vi "Daq_withRPM.vi"() -> ()   [LabVIEW 2019]
panel:
  in  "Salvar Ensaio":path
  out "RPM Atual":i32
  in  "Tempo de transição (s)":u32=2000
  out "Running":bool=TRUE
  in  "Parar Ensaio":bool
  in  "Tempo por RPM (min)":dbl
  in  "configuração de porta":T1={"Serial VCC"="", "timeout"=2, "baud rate"=600, "flow control"=0, "data bits"=8, "parity"=enum."None", "stop bits"=10, "termination char"=FALSE} {"stop bits" items=["1.0"=10, "1.5"=15, "2.0"=20]; "flow control" items=["None", "XON/XOFF", "RTS/CTS", "XON/XOFF & RTS/CTS", "DTR/DSR", "XON/XOFF & DTR/DSR"]}
  out "Grafico Aceleração":dynamicdata(graph)
  in  "Start button":bool
  in  "Passo de RPM":i32
  in  "Máximo RPM":i32
  in  "Mínimo RPM":i32
  # "Ensaio de Vibração"
  # "Configuração"
  # "Rodando"
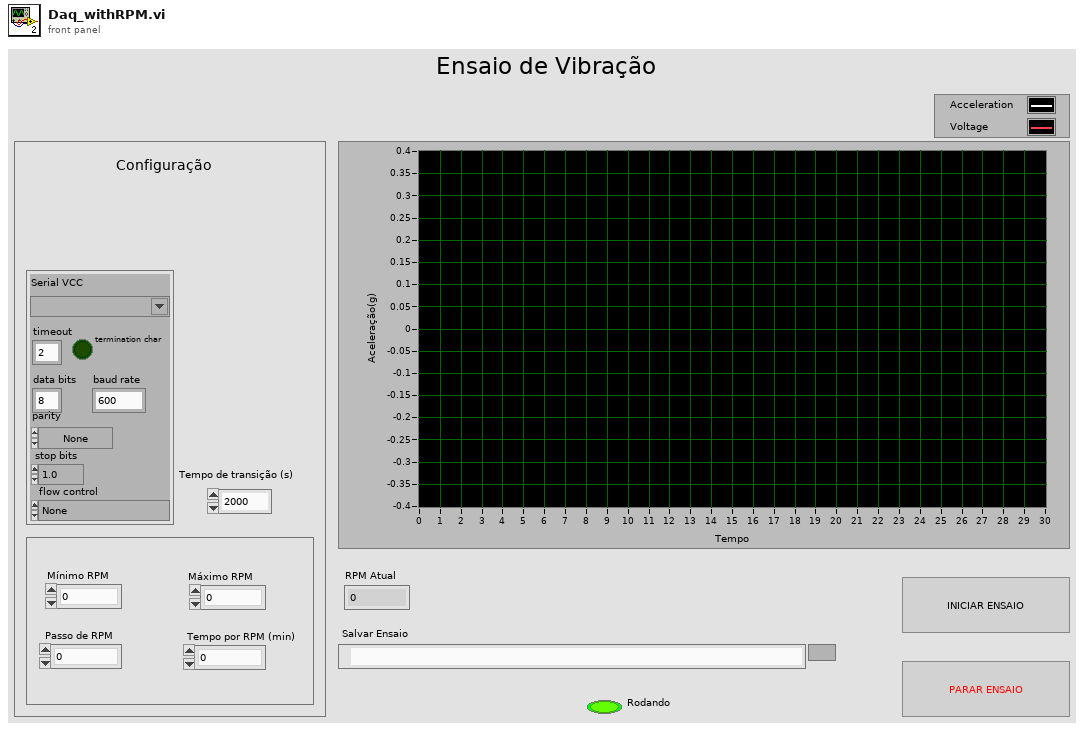
[diagram p1: front panel]
types:
  T1 = cluster{"Serial VCC":refnum<visa-resource-name>, "timeout":u32, "baud rate":u32, "flow control":u16, "data bits":u16, "parity":enum16{"None", "Odd", "Even", "Mark", "Space"}, "stop bits":u16, "termination char":bool}
  T2 = enum16{"Start Comm.", "End Comm.", "Wait", "Send Static Message", "Set Speed", "Set PWM Mode", "Set PWM Frequency"}
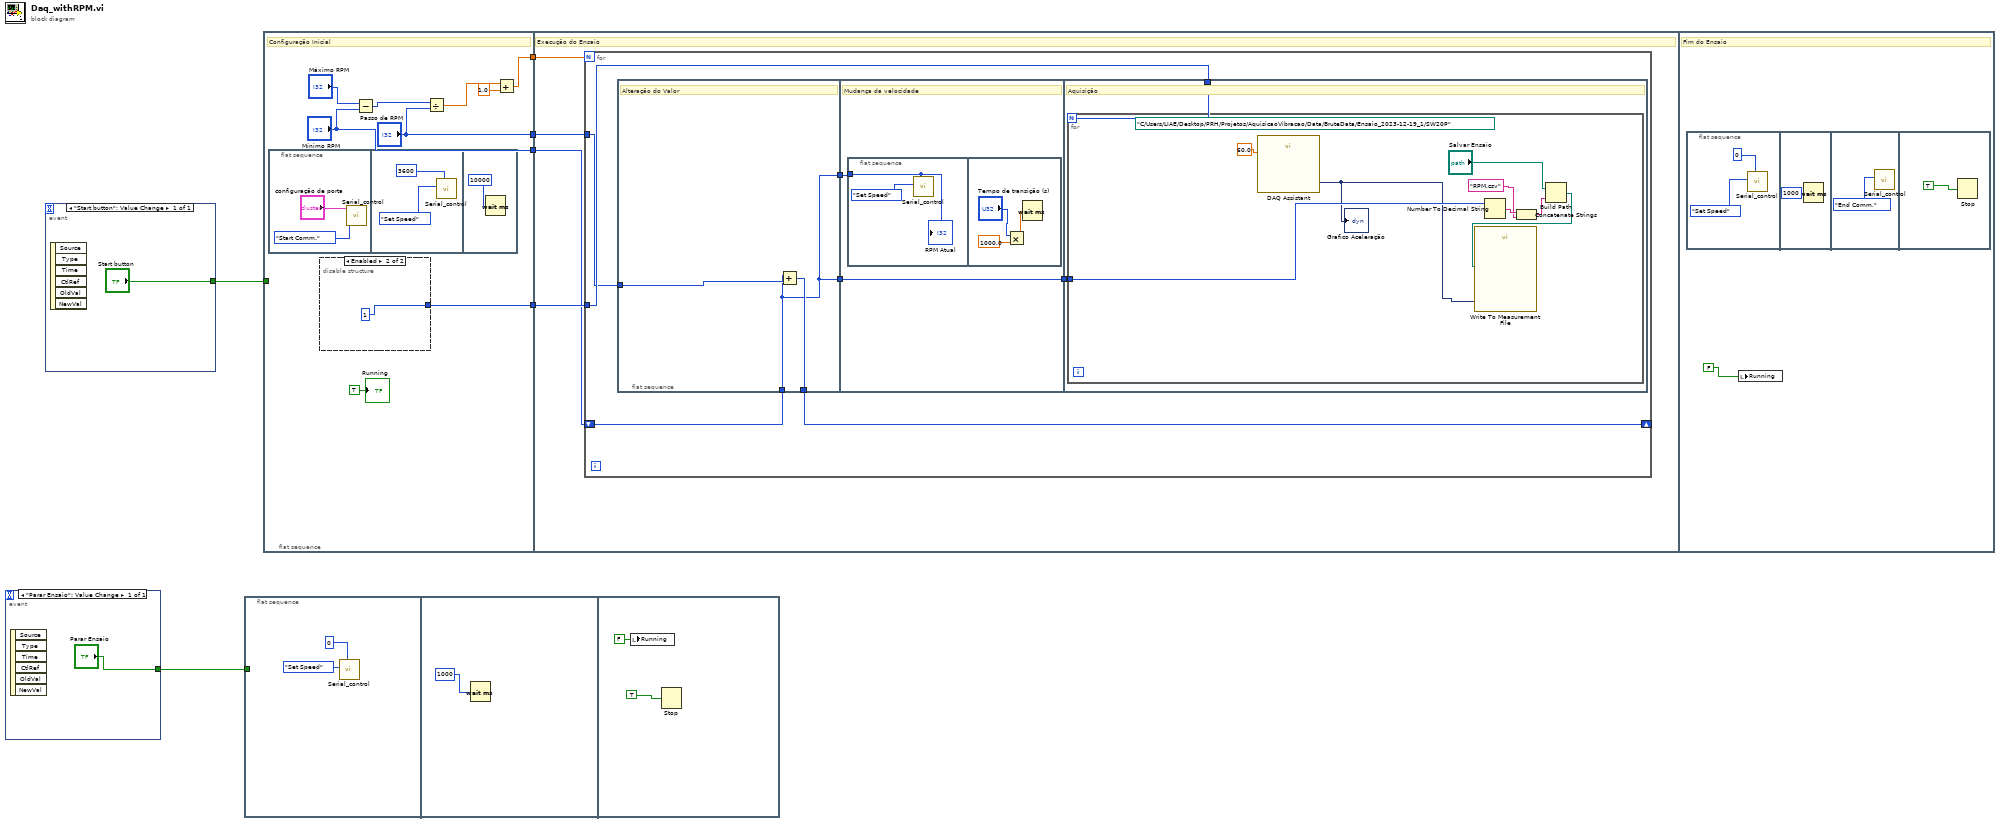
[diagram p0: block diagram]
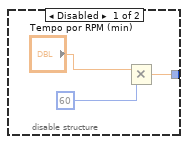
[diagram p2: hidden frame]
diagram:
  n1 = event shown="[0] \"Parar Ensaio\": Value Change" {
    selector: _ -> [_]
    dyn-events: _ -> [_]
    timeout: _ -> [_]
    tunnel: ["Parar Ensaio"] -> w2
    event "Parar Ensaio": Value Change {
      n2 = event-data() -> ()  [unwired: 1 in, 6 out]
    }
  }
  n3 = event shown="[0] \"Start button\": Value Change" {
    selector: _ -> [_]
    dyn-events: _ -> [_]
    timeout: _ -> [_]
    tunnel: ["Start button"] -> w6
    event "Start button": Value Change {
      n4 = event-data() -> ()  [unwired: 1 in, 6 out]
    }
  }
  n5 = flat-sequence {
    tunnel: w2 -> [_]
    frame #0 {
      n6 = call "Serial_control.vi"("Enviar número"=u16 0, "Função"=T2."Set Speed") -> ()  [unwired: 3 in, 4 out]
    }
    frame #1 {
      n7 = Wait (ms)(milliseconds to wait=u32 1000 ("millisecond timer value")) -> ()  [unwired: 1 out]
    }
    frame #2 {
      n8 = local write "Running"(FALSE ("Running")) -> ()
      n9 = Stop(stop? (T)=TRUE) -> ()
    }
  }
  n10 = flat-sequence {
    tunnel: w6 -> [_]
    tunnel: ["Passo de RPM"] -> w5
    tunnel: [w19] -> w4
    tunnel: ["Mínimo RPM"] -> w3
    tunnel: [w14] -> w1
    tunnel: w5 -> [w35]
    tunnel: w4 -> [w34]
    tunnel: w3 -> [w33]
    tunnel: w1 -> [w32]
    frame #0 {
      # "Configuração Inicial"
      n11 = flat-sequence {
        frame #0 {
          n12 = call "Serial_control.vi"("Função"=T2."Start Comm.", "comm cluster"="configuração de porta") -> ()  [unwired: 3 in, 4 out]
        }
        frame #1 {
          n13 = call "Serial_control.vi"("Enviar número"=u16 3600, "Função"=T2."Set Speed") -> ()  [unwired: 3 in, 4 out]
        }
        frame #2 {
          n14 = Wait (ms)(milliseconds to wait=u32 10000) -> ()  [unwired: 1 out]
        }
      }
      n15 = disable-structure shown="Enabled" {
        disable-tunnel: [w28 1] -> w19
        frame Disabled {
          n16 = Multiply(x="Tempo por RPM (min)", y=60) -> (x*y=w28:dbl)
        }
        frame Enabled {
        }
      }
      n17 = Subtract(x="Máximo RPM", y="Mínimo RPM") -> (x-y=w21:i32)
      n18 = Divide(x=w21, y="Passo de RPM") -> (x/y=w16:dbl)
      n19 = Add(x=w16, y=1.0) -> (x+y=w14:dbl)
      "Running" <- TRUE
    }
    frame #1 {
      # "Execução do Ensaio"
      n20 = for {
        N: w32 -> [_]
        shift-right: [w39] -> _
        shift-left: w33 -> [w40]
        tunnel: w35 -> [w41]
        tunnel: w34 -> [w42]
        n21 = flat-sequence {
          tunnel: w41 -> [w45]
          tunnel: w40 -> [w43]
          tunnel: [w44] -> w39
          tunnel: [w43] -> w37
          tunnel: [w43] -> w36
          tunnel: [w47] -> w38
          tunnel: w37 -> [w47]
          tunnel: w36 -> [w46]
          tunnel: w42 -> [w54]
          tunnel: w38 -> [w53]
          frame #0 {
            # "Alteração do Valor"
            n22 = Add(x=w43, y=w45) -> (x+y=w44:i32)
          }
          frame #1 {
            # "Mudança da velocidade"
            n23 = flat-sequence {
              tunnel: w46 -> [w48]
              frame #0 {
                n24 = call "Serial_control.vi"("Enviar número"=w48, "Função"=T2."Set Speed") -> ()  [unwired: 3 in, 4 out]
                "RPM Atual" <- w48
              }
              frame #1 {
                n25 = Multiply(x="Tempo de transição (s)", y=1000.0) -> (x*y=w52:dbl)
                n26 = Wait (ms)(milliseconds to wait=w52) -> ()  [unwired: 1 out]
              }
            }
          }
          frame #2 {
            # "Aquisição"
            n27 = for {
              N: w54 -> [_]
              tunnel: w53 -> [w61]
              (unwired) path "C:/Users/LIAE/Desktop/PRH/Projetos/AquisicaoVibracao/Data/BruteData/Ensaio_2023-12-19_1/SW20P" ("base path")
              n28 = call "DAQ Assistant"("timeout (s)"=60.0) -> ("data"=w59:dynamicdata)  [unwired: 15 in, 3 out]
              "Grafico Aceleração" <- w59
              n29 = Number To Decimal String(number=w61) -> (decimal integer string=w58:string)  [unwired: 1 in]
              n30 = Concatenate Strings(w58, "RPM.csv" ("name or relative path")) -> (w56:string)
              n31 = Build Path(base path="Salvar Ensaio", name or relative path=w56) -> (appended path=w60:path)
              n32 = call "Write To Measurement File"("Signals"=w59, "Filename"=w60) -> ()  [unwired: 15 in, 3 out]
            }
          }
        }
      }
    }
    frame #2 {
      # "Fim do Ensaio"
      n33 = flat-sequence {
        frame #0 {
          n34 = call "Serial_control.vi"("Enviar número"=u16 0, "Função"=T2."Set Speed") -> ()  [unwired: 3 in, 4 out]
        }
        frame #1 {
          n35 = Wait (ms)(milliseconds to wait=u32 1000) -> ()  [unwired: 1 out]
        }
        frame #2 {
          n36 = call "Serial_control.vi"("Função"=T2."End Comm.") -> ()  [unwired: 4 in, 4 out]
        }
        frame #3 {
          n37 = Stop(stop? (T)=TRUE) -> ()
        }
      }
      n38 = local write "Running"(FALSE) -> ()
    }
  }
